vi "evaluateZeroDrift.vi"(6 "chIndex":i32, 7 "Traverse line In":T3 {"Carrier_2 Q (l/min)" format="%#.2f"; "Row Duration (mins)" format="%#.1f"; "Row No" min=0; "Trace Gas Concentration (%)" min=0.0 format="%#_4f"; "Carrier_1 Q (l/min)" format="%#.4f"; "Start X" format="%#.2f"; "Start Y" format="%#.2f"; "Start Z" format="%#.2f"; "End X" format="%#.2f"; "End Y" format="%#.2f"; "End Z" format="%#.2f"; "Tunnel Speed" format="%#.2f"; "Averaging time (mins)" min=0.0 format="%#.2f"}, 9 "Time Trace":T1, 10 "Inst type":T2, 11 "Inst name":string) -> (1 "Drifty?":bool, 2 "ratio":dbl, 3 "tableRow":string[](array[string]))   [LabVIEW 2022 SP3]
uses:
  Gen Trav/Traverse_cluster.ctl
  Gen Trav/Spacing.ctl
  Controls/Multi_run_mode.ctl
  Controls/Inst_type.ctl
  Controls/Time_Trace_Cluster.ctl
  <vilib>/Analysis/NI_AALPro.lvlib
  <vilib>/Analysis/NI_AALBase.lvlib
panel:
  # "X           Y          Z"
  # "Start"
  # "End"
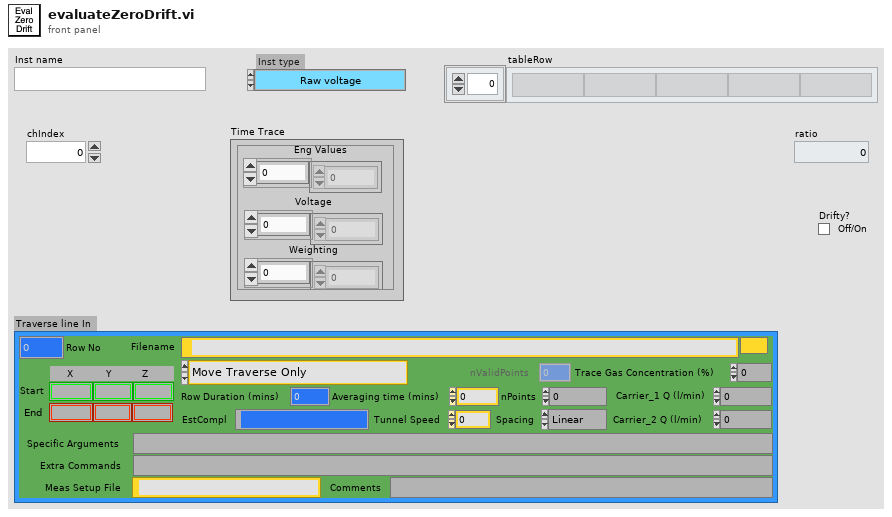
[diagram p1: front panel]
types:
  T1 = typedef "Time_Trace_Cluster.ctl" = cluster{"Weighting":dbl[], "Voltage":dbl[], "Eng Values":dbl[]}
  T2 = typedef "Inst_type.ctl" = enum16{"Raw voltage", "Raw with zero offsetting", "Propeller anemometer", "Pressure Transducer", "Pitot-static tube", "Hot wire", "Cross wire 1", "Cross wire 2", "Generic Linear", "Generic Polynomial", "Generic BackPoly", "Fast FID", "Thermocouple", "Cold wire", "Pulsed Wire", "LDA Vel", "LDA Tran time", "LDA Arr time", "Microphone"}
  T3 = typedef "Traverse_cluster.ctl" = cluster{"Start X":sgl, "Start Y":sgl, "Start Z":sgl, "End X":sgl, "End Y":sgl, "End Z":sgl, "nPoints":i32, "Spacing":T4, "Filename":path, "Tunnel Speed":dbl, "Averaging time (mins)":dbl, "Extra Commands":string, "Carrier_1 Q (l/min)":dbl, "Carrier_2 Q (l/min)":dbl, "Trace Gas Concentration (%)":dbl, "Specific Arguments":string, "Comments":string, "Row No":i32, "Row Type Selector":T5, "EstCompl":string, "Row Duration (mins)":dbl, "nValidPoints":i32, "Meas Setup File":string}
  T4 = typedef "Spacing.ctl" = enum16{"Linear", "Log", "Gauss", "Specified", "N/A"}
  T5 = typedef "Multi_run_mode.ctl" = enum16{"Move Traverse Only", "Set Tunnel Speed Only", "Set Source Only", "Set Measurement Conditions", "Single Measurement", "Vertical Profile", "Lateral Profile", "Longitudinal Profile", "Multi-Axis Profile", "Explore Volume", "Auto Calibrate", "Meas Fast FID Bkgnd", "Check Beam Power", "Scanning Valve Measurement", "Run VI Named:", "Set ADAM Ch", "Wait (minutes)", "Send Message", "Synchronize With:", "Fall Back to this Row", "Turn Off Row Repeating", "Traverse 3D Volume", "Blank Row", "Jump to Fall Back Row"}
  T6 = typedef "Data for Inst Type.ctl" = enum16{"Eng Values", "Voltage"}
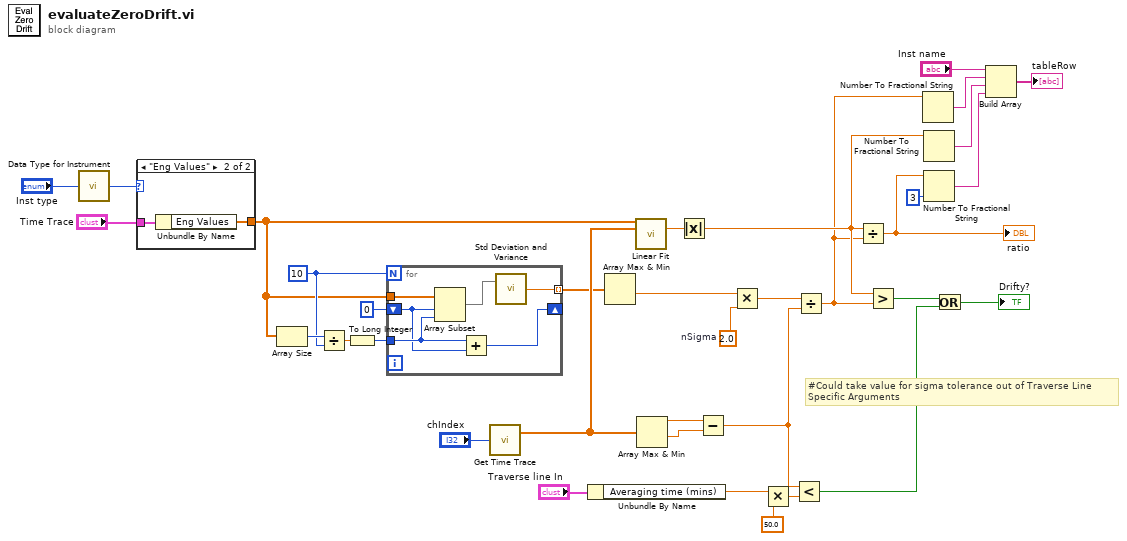
[diagram p0: block diagram]
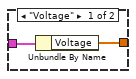
[diagram p2: hidden frame]
diagram:
  w15 = 2.0  # nSigma
  w8 = 10 ("y")
  # "#Could take value for sigma tolerance out of Traverse Line\nSpecific Arguments"
  n1 = call "Data Type for Instrument.vi"("Inst type"="Inst type") -> ("Data for Inst Type"=w29:T6)
  n2 = case shown="\"Eng Values\"" w29 {
    tunnel: [w37 w39] -> w4
    tunnel: "Time Trace" -> [w36 w38]
    frame "Voltage" {
      n3 = Unbundle By Name(w36) -> ("Voltage"=w37:dbl[])
    }
    frame "Eng Values" {
      n4 = Unbundle By Name(w38) -> ("Eng Values"=w39:dbl[])
    }
  }
  n5 = Array Size(array=w4) -> (size(s)=w12:i32)
  n6 = Divide(x=w12, y=w8) -> (x/y=w10:dbl)
  n7 = To Long Integer(number=w10) -> (32bit integer=w9:i32)
  n8 = for {
    N: w8 -> [_]
    tunnel: w4 -> [w45]
    shift-right: [w42] -> _
    shift-left: 0 ("y") -> [w43]
    tunnel: w9 -> [w44]
    tunnel: [w40] -> w7 mode=indexing
    n9 = Array Subset(array=w45, index=w43, length=w44) -> (w41:dbl[])
    n10 = Add(x=w44, y=w43) -> (x+y=w42:i32)
    n11 = call <vilib>:"Std Deviation and Variance.vi"("X"=w41) -> ("standard deviation"=w40:dbl)  [unwired: 1 in, 2 out]
  }
  n12 = call "Get Time Trace.vi"("Channel Index"="chIndex") -> ("Time (s)"=w31:dbl[])  [unwired: 1 out]
  n13 = Unbundle By Name("Traverse line In") -> ("Averaging time (mins)"=w32:dbl)
  n14 = Array Max & Min(array=w7) -> (min value=w2:dbl)  [unwired: 3 out]
  n15 = call <vilib>:"Linear Fit.vi"("Y"=w4, "X"=w31) -> ("slope"=w13:dbl)  [unwired: 9 in, 4 out]
  n16 = Array Max & Min(array=w31) -> (max value=w6:dbl, min value=w5:dbl)  [unwired: 2 out]
  n17 = Absolute Value(x=w13) -> (abs(x)=w18:dbl)
  n18 = Subtract(x=w6, y=w5) -> (x-y=w24:dbl)
  n19 = Multiply(x=w2, y=w15) -> (x*y=w1:dbl)
  n20 = Multiply(x=w32, y=50.0) -> (x*y=w35:dbl)
  n21 = Less?(x=w24, y=w35) -> (x < y?=w26:bool)
  n22 = Divide(x=w1, y=w24) -> (x/y=w3:dbl)
  n23 = Divide(x=w18, y=w3) -> (x/y=w21:dbl)
  "ratio" <- w21
  n24 = Greater?(x=w18, y=w3) -> (0:w25:bool)
  n25 = Number To Fractional String(number=w3) -> (F-format string=w17:string)  [unwired: 3 in]
  n26 = Number To Fractional String(number=w18) -> (F-format string=w19:string)  [unwired: 3 in]
  n27 = Number To Fractional String(number=w21, precision (6)=i16 3) -> (F-format string=w22:string)  [unwired: 2 in]
  n28 = Or(x=w25, y=w26) -> (x .or. y?=→"Drifty?":bool)
  n29 = Build Array("Inst name", w17, w19, w22) -> (→"tableRow":string[])
